vi "sub_select_measurement_or_simulation.vi"() -> ()   [LabVIEW 2013]
panel:
  out "참 버튼?":bool
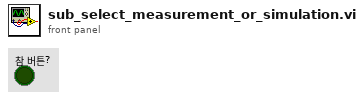
[diagram p1: front panel]
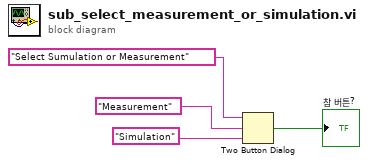
[diagram p0: block diagram]
diagram:
  n1 = Two Button Dialog(message="Select Sumulation or Measurement" ("메시지"), 1:"Simulation" ("참 버튼 이름(\"확인\")"), 2:"Measurement" ("거짓 버튼 이름(\"취소\")")) -> (T button?=→"참 버튼?":bool)
